vi "WriteOverlayColor.vi"(8 "error in":errorcluster, 10 "Colors":T1[](array[typedef]), 11 "Image Reference In":T2) -> (0 "error out":errorcluster, 3 "Image Reference Out":T2)   [LabVIEW 2024, in "OpenLvVision_Overlays.lvlib"]
doc: "Writes the overlay color for an group."
uses:
  OpenLvVision_Overlays.lvlib
  <vilib>/OpenLvVision/OpenLvVision_Image/Management/TypeDef/OLV Image.ctl
  TypeDefs/ColorGroup.ctl
  <vilib>/OpenLvVision/OpenLvVision_Image/Management/OLV Management.lvlib
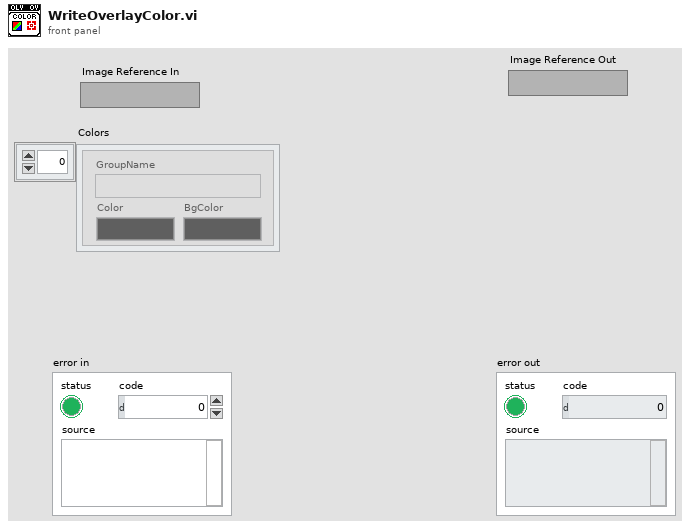
[diagram p1: front panel]
types:
  T1 = typedef "OpenLvVision_Overlays.lvlib/ColorGroup.ctl" = cluster{"GroupName":string, "Color":u32, "BgColor":u32}
  T2 = typedef "OLV OpenLvVision_Image.lvlib/OLV Management.lvlib/OLV Image.ctl" = refnum<image>
  T3 = typedef "IMAQ Image.ctl" = refnum<image>
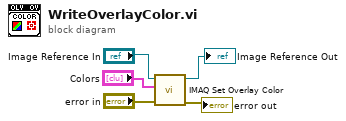
[diagram p0: block diagram]
diagram:
  n1 = call "IMAQ Set Overlay Color"("error in (no error)"="error in", "Colors"="Colors", "Image"="Image Reference In") -> ("error out"=→"error out":errorcluster, "Image Out"=→"Image Reference Out":T3)  [unwired: 7 in]
